vi "fit_cuts.vi"(9 "Array":dbl[](array[numeric]), 10 "Intensity Graph":dbl[][](graph)) -> (2 "Waveform Graph":dbl[][](graph))   [LabVIEW 2016]
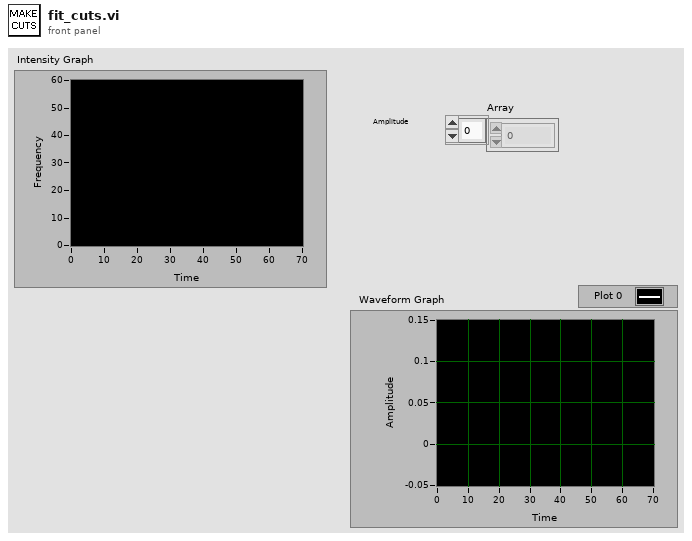
[diagram p1: front panel]
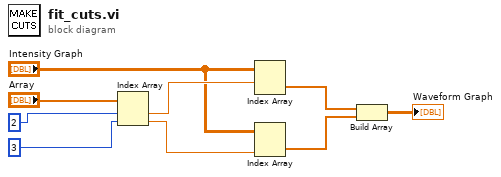
[diagram p0: block diagram]
diagram:
  n1 = Index Array(array="Array", index #1=2, index #2=3) -> (element #1=w6:dbl, element #2=w5:dbl)
  n2 = Index Array(array="Intensity Graph", index (row)=w6) -> (element=w2:dbl[])  [unwired: 1 in]
  n3 = Index Array(array="Intensity Graph", index (col)=w5) -> (element=w3:dbl[])  [unwired: 1 in]
  n4 = Build Array(w2, w3) -> (→"Waveform Graph":dbl[][])
